vi "NewE2E_AnalyserTester.vi"() -> ()   [LabVIEW 2014]
uses:
  TypeDef_AnalyserActions.ctl
panel:
  out "NewVal 2":dbl
  out "NewVal":dbl
  out "Received 2":string
  out "Received":string
  in  "Stop Button":bool
  in  "A2 Set Voltages":T1={"RE"=0.0, "LE"=0.0, "DX"=-11.0, "DY"=-11.0, "AM"=0.0, "IH"=5.0, "OH"=5.0}
  out "A2 Measured Voltages":T1={"RE"=0.0, "LE"=0.0, "DX"=-11.0, "DY"=-11.0, "AM"=0.0, "IH"=5.0, "OH"=5.0}
  out "A1 Measured Voltages":T1={"RE"=0.0, "LE"=0.0, "DX"=-11.0, "DY"=-11.0, "AM"=0.0, "IH"=5.0, "OH"=5.0}
  in  "A1 Set Voltages":T1={"RE"=0.0, "LE"=0.0, "DX"=-11.0, "DY"=-11.0, "AM"=0.0, "IH"=5.0, "OH"=5.0}
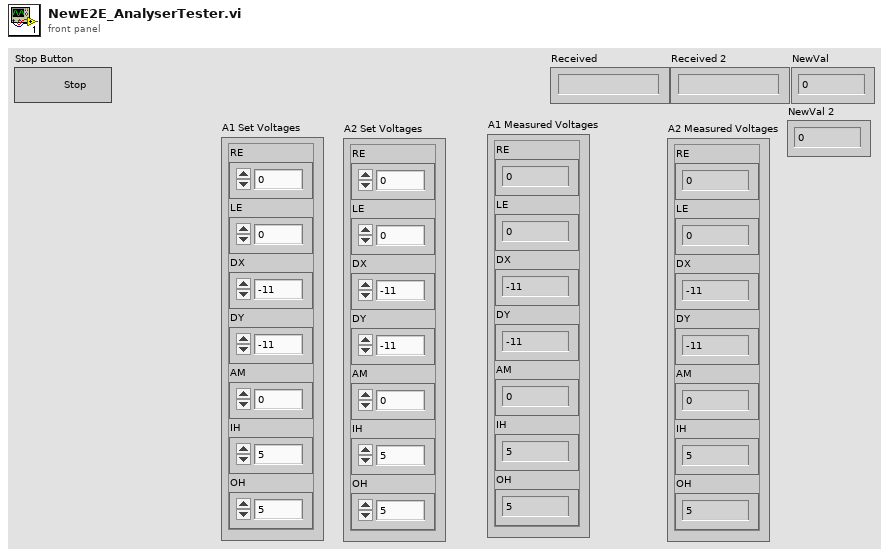
[diagram p1: front panel]
types:
  T1 = cluster{"RE":dbl, "LE":dbl, "DX":dbl, "DY":dbl, "AM":dbl, "IH":dbl, "OH":dbl}
  T2 = typedef "TypeDef_AnalyserActions.ctl" = enum16{"Find COM Port", "Find & Connect", "Connect Port", "Disconnect Port", "Enable Checksum", "Disable Checksum", "Get ID", "Msg & ACKNAK", "Msg & Response", "Set RE Voltage", "Set LE Voltage", "Set DX Voltage", "Set DY Voltage", "Set AM Voltage", "Set IH Voltage", "Set OH Voltage", "Get AE", "Get RE", "Get LE", "Get DX", "Get DY", "Get AM", "Get IH", "Get OH"}
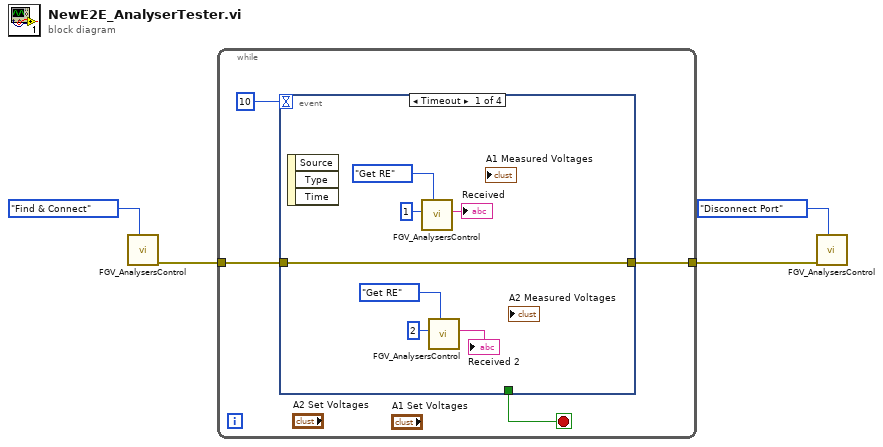
[diagram p0: block diagram]
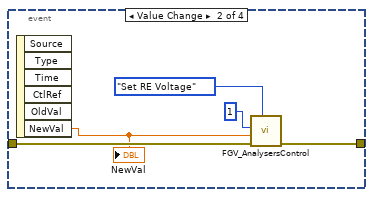
[diagram p2: hidden frame]
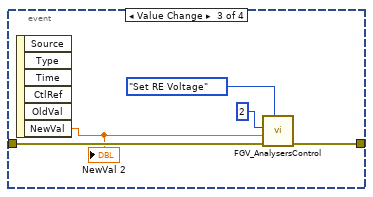
[diagram p3: hidden frame]
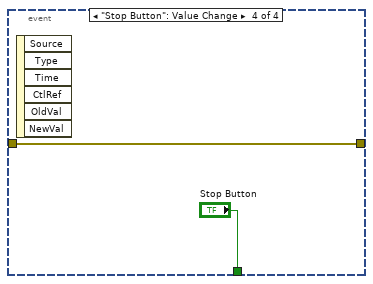
[diagram p4: hidden frame]
diagram:
  n1 = call "FGV_AnalysersControl.vi"("Action"=TypeDef_AnalyserActions."Find & Connect") -> ("error out"=w2:errorcluster)  [unwired: 8 in, 2 out]
  n2 = while {
    tunnel: w2 -> [w5]
    tunnel: [w6] -> w1
    stop <- w7 stop-if-true
    n3 = event shown="[0] Timeout" {
      selector: _ -> [_ _ _ _]
      dyn-events: _ -> [_ _ _ _]
      timeout: 10 -> [_ _ _ _]
      tunnel: [_ _ _ "Stop Button"] -> w7
      tunnel: [w15 w19 w22 w26] -> w6
      tunnel: w5 -> [w15 w18 w23 w26]
      event Timeout {
        n4 = event-data() -> ()  [unwired: 1 in, 3 out]
        n5 = call "FGV_AnalysersControl.vi"("Action"=TypeDef_AnalyserActions."Get RE", "Analyser"=1) -> ("Received"=→"Received":string)  [unwired: 7 in, 2 out]
        n6 = call "FGV_AnalysersControl.vi"("Action"=TypeDef_AnalyserActions."Get RE", "Analyser"=2) -> ("Received"=→"Received 2":string)  [unwired: 7 in, 2 out]
      }
      event "A1 Set Voltages.RE": Value Change {
        n7 = event-data() -> ("NewVal"=w17:dbl)  [unwired: 1 in, 5 out]
        "NewVal" <- w17
        n8 = call "FGV_AnalysersControl.vi"("Action"=TypeDef_AnalyserActions."Set RE Voltage", "Error In"=w18, "Set Voltage"=w17, "Analyser"=1) -> ("error out"=w19:errorcluster)  [unwired: 5 in, 2 out]
      }
      event "A2 Set Voltages.RE": Value Change {
        n9 = event-data() -> ("NewVal"=w21:dbl)  [unwired: 1 in, 5 out]
        "NewVal 2" <- w21
        n10 = call "FGV_AnalysersControl.vi"("Action"=TypeDef_AnalyserActions."Set RE Voltage", "Error In"=w23, "Set Voltage"=w21, "Analyser"=2) -> ("error out"=w22:errorcluster)  [unwired: 5 in, 2 out]
      }
      event "Stop Button": Value Change {
        n11 = event-data() -> ()  [unwired: 1 in, 6 out]
      }
    }
  }
  n12 = call "FGV_AnalysersControl.vi"("Action"=TypeDef_AnalyserActions."Disconnect Port", "Error In"=w1) -> ()  [unwired: 7 in, 3 out]
